vi "dfd_Check Input (2D).vi"(8 "error in (no error)":errorcluster, 10 "number of bands":i32, 11 "x":dbl[][](array[numeric])) -> (0 "error out":errorcluster, 3 "dup x":dbl[][](array[numeric]))   [LabVIEW 2017, in "NI_DigFilter_FilterBank.lvlib"]
uses:
  <vilib>/addons/Digital Filter Design/NI_DigFilter_FilterBank.lvlib
  <vilib>/addons/Digital Filter Design/_Misc.llb/dfd_Error Handlers (Single).vi
  <vilib>/addons/Digital Filter Design/NI_DigFilterLicensed.lvlib
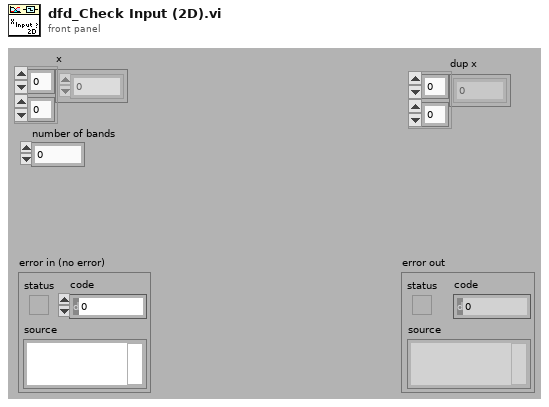
[diagram p1: front panel]
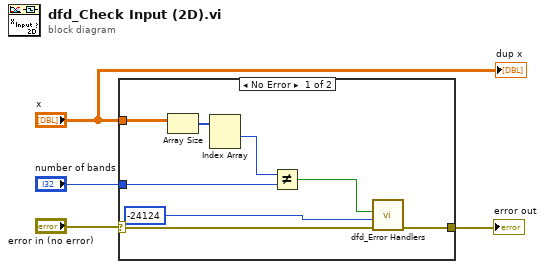
[diagram p0: block diagram]
diagram:
  n1 = case shown="No Error" "error in (no error)" {
    selector: "error in (no error)" -> [w8 w13]
    tunnel: [w5 w13] -> w3
    tunnel: "x" -> [w6 _]
    tunnel: "number of bands" -> [w10 _]
    frame No Error {
      n2 = Array Size(array=w6) -> (size(s)=w12:i32[])
      n3 = Index Array(array=w12) -> (element #1=w11:i32)  [unwired: 2 in, 1 out]
      n4 = Not Equal?(x=w11, y=w10) -> (x != y?=w7:bool)
      n5 = call-poly <vilib>:"dfd_Error Handlers.vi"("error in (no error)"=w8, "error code"=-24124 ("ERR_#SIGNALS_INCONSISTENT_#BAND"), "condition failed?"=w7) -> ("error out"=w5:errorcluster)  [unwired: 8 in]
    }
    frame Error {
    }
  }
  "error out" <- w3
  "dup x" <- "x"
